vi "SCP Upload File.vi"(8 "Error In":errorcluster, 9 "Target Directory":string="/home/debian/", 10 "Local File":path, 11 "SCP Session":refnum<k24>) -> (0 "Error Out":errorcluster, 3 "SCP Session":refnum<k24>)   [LabVIEW 2014, in "LMH-LINX.lvlib"]
uses:
  <vilib>/MakerHub/LINX/LMH-LINX.lvlib
  C:/Program Files (x86)/National Instruments/LabVIEW 2014/vi.lib/MakerHub/LINX/Resources/Renci.SshNet.dll
  Resources/Renci.SshNet.dll
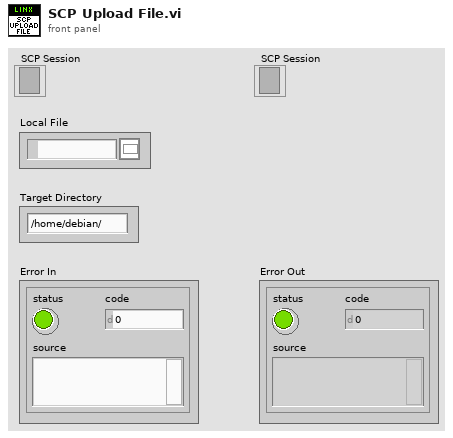
[diagram p1: front panel]
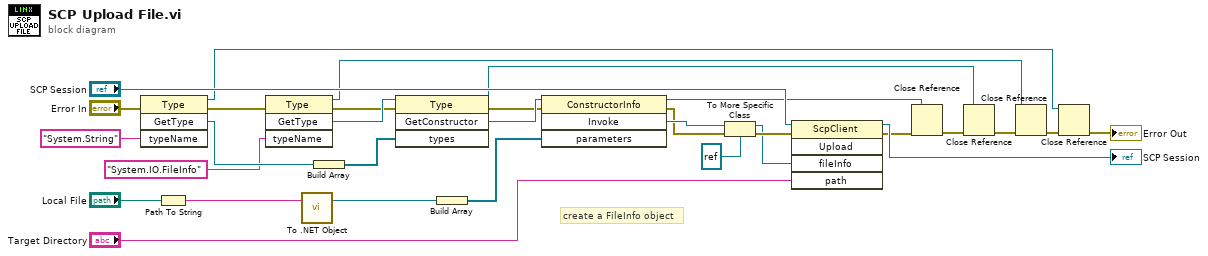
[diagram p0: block diagram]
diagram:
  # "create a FileInfo object"
  n1 = invoke class="Type" method="GetType"(error in="Error In", "typeName"="System.String") -> (reference out=w2:refnum<k24>, error out=w13:errorcluster, "GetType"=w19:refnum<k24>)  [unwired: 2 in, 1 out]
  n2 = Path To String(path="Local File") -> (string=w31:string)
  n3 = invoke class="Type" method="GetType"(error in=w13, "typeName"="System.IO.FileInfo") -> (reference out=w4:refnum<k24>, error out=w12:errorcluster, "GetType"=w17:refnum<k24>)  [unwired: 2 in, 1 out]
  n4 = call <vilib>:"To .NET Object.vi"("anything"=w31) -> (".NET object"=w22:refnum<k24>)  [unwired: 1 in, 1 out]
  n5 = Build Array(w19) -> (w21:refnum<k24>[])
  n6 = invoke class="Type" method="GetConstructor"(reference=w17, error in=w12, "types"=w21) -> (reference out=w5:refnum<k24>, error out=w11:errorcluster, "GetConstructor"=w20:refnum<k24>)  [unwired: 1 in, 1 out]
  n7 = Build Array(w22) -> (w23:refnum<k24>[])
  n8 = invoke class="ConstructorInfo" method="Invoke"(reference=w20, error in=w11, "parameters"=w23) -> (reference out=w8:refnum<k24>, error out=w10:errorcluster, "Invoke"=w25:refnum<k24>)  [unwired: 1 in, 1 out]
  n9 = To More Specific Class(target class=refnum<k24> refnum ("fileInfo"), reference=w25, error in=w10) -> (specific class reference=w26:refnum<k24>, error out=w28:errorcluster)
  n10 = invoke class="ScpClient" method="Upload"(reference="SCP Session", error in=w28, "fileInfo"=w26, "path"="Target Directory") -> (reference out=→"SCP Session":refnum<k24>, error out=w9:errorcluster)  [unwired: 1 in, 3 out]
  n11 = Close Reference(reference=w8, error in (no error)=w9) -> (error out=w7:errorcluster)
  n12 = Close Reference(reference=w5, error in (no error)=w7) -> (error out=w6:errorcluster)
  n13 = Close Reference(reference=w4, error in (no error)=w6) -> (error out=w3:errorcluster)
  n14 = Close Reference(reference=w2, error in (no error)=w3) -> (error out=→"Error Out":errorcluster)
